vi "446x_AI_MinMax.vi"(2 "446x AI":T1) -> (6 "AI.Min":dbl, 7 "AI.Max":dbl)   [LabVIEW 2016, in "UI_DAQ_config.lvclass"]
uses:
  UI_DAQ_config.lvclass
  Typedefs/446xAI-enum.ctl
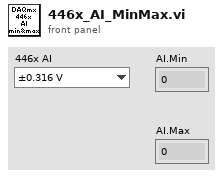
[diagram p1: front panel]
types:
  T1 = typedef "UI_DAQ_config.lvclass/446xAI-enum.ctl" = enum16{"±0.316 V", "±1.00 V", "±3.16 V", "±10.0 V", "±31.6 V", "±42.4 V"}
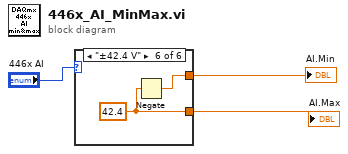
[diagram p0: block diagram]
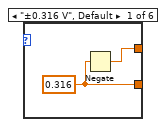
[diagram p2: hidden frame]
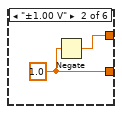
[diagram p3: hidden frame]
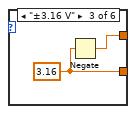
[diagram p4: hidden frame]
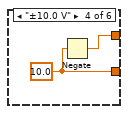
[diagram p5: hidden frame]
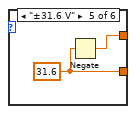
[diagram p6: hidden frame]
diagram:
  n1 = case shown="\"±42.4 V\"" "446x AI" {
    tunnel: [w4 w6 w8 w10 w12 w14] -> w2
    tunnel: [w5 w7 w9 w11 w13 w15] -> w1
    frame "±0.316 V", Default {
      w5 = 0.316 ("AI.Min")
      n2 = Negate(x=w5) -> (-x=w4:dbl)
    }
    frame "±1.00 V" {
      w7 = 1.0 ("AI.Min")
      n3 = Negate(x=w7) -> (-x=w6:dbl)
    }
    frame "±3.16 V" {
      w9 = 3.16 ("AI.Min")
      n4 = Negate(x=w9) -> (-x=w8:dbl)
    }
    frame "±10.0 V" {
      w11 = 10.0 ("AI.Min")
      n5 = Negate(x=w11) -> (-x=w10:dbl)
    }
    frame "±31.6 V" {
      w13 = 31.6 ("AI.Min")
      n6 = Negate(x=w13) -> (-x=w12:dbl)
    }
    frame "±42.4 V" {
      w15 = 42.4 ("AI.Min")
      n7 = Negate(x=w15) -> (-x=w14:dbl)
    }
  }
  "AI.Min" <- w2
  "AI.Max" <- w1
